vi "FL_Reshape_data_back_for_saving.vi"(9 "Read frame size":u32=8, 11 "DEC SGL input":sgl[](array[numeric])) -> (3 "DEC SGL Output":sgl[][](array[numeric]))   [LabVIEW 2018, in "Tracker.lvlib"]
uses:
  Tracker.lvlib
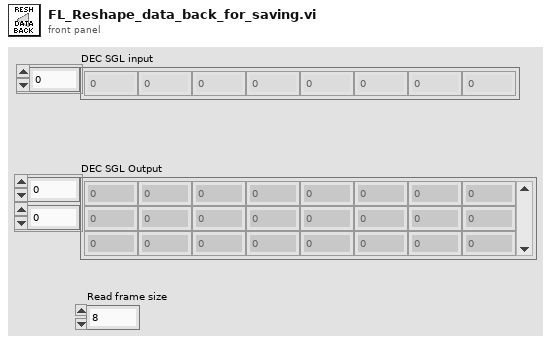
[diagram p1: front panel]
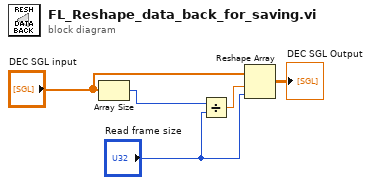
[diagram p0: block diagram]
diagram:
  n1 = Array Size(array="DEC SGL input") -> (size(s)=w1:i32)
  n2 = Divide(x=w1, y="Read frame size") -> (x/y=w4:dbl)
  n3 = Reshape Array("DEC SGL input", w4, "Read frame size") -> (→"DEC SGL Output":sgl[][])
